vi "displayTest.vi"() -> ()   [LabVIEW 2010]
panel:
  in  "output cluster":T1
  out "display":T2={"电压/V"=[220.214842, 220.567942, 0.0], "测量变量显示"={"number: 0 to 1"=0.0, "number: 0 to 1"=0.0, "number: 0 to 1"=0.0}, "测量变量显示 2"={"number: 0 to 1"=0.0, "number: 0 to 1"=0.0, "number: 0 to 1"=0.0}}
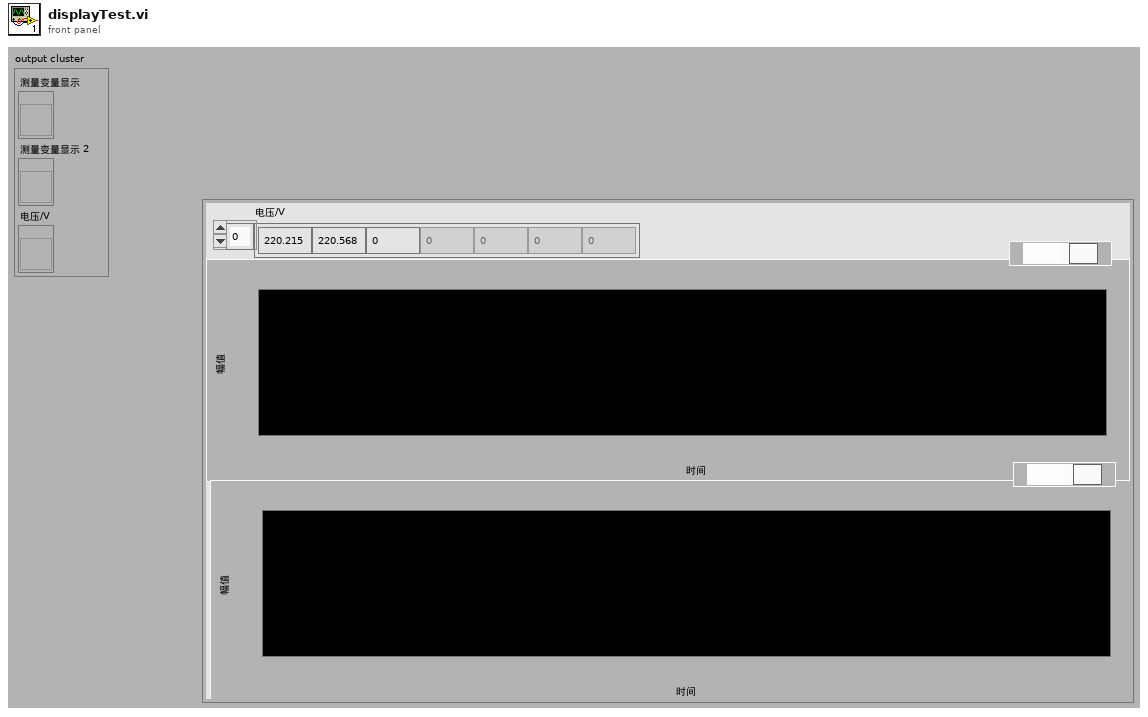
[diagram p1: front panel]
types:
  T1 = cluster{"测量变量显示":refnum<vi>, "测量变量显示 2":refnum<vi>, "电压/V":refnum<vi>}
  T2 = cluster{"电压/V":dbl[], "测量变量显示":cluster{"number: 0 to 1":dbl, "number: 0 to 1":dbl, "number: 0 to 1":dbl}, "测量变量显示 2":cluster{"number: 0 to 1":dbl, "number: 0 to 1":dbl, "number: 0 to 1":dbl}}
  T3 = cluster{"number: 0 to 1":dbl, "number: 0 to 1":dbl, "number: 0 to 1":dbl}[]
  T4 = typedef "OutputDataFormat.ctl" = cluster{"property":string, "dataIdentity":string, "value":string, "address":string, "timeStamp":string, "unit":string, "numID":i32, "VarableID":T5}
  T5 = typedef "VarableID.ctl" = enum16{"current", "power", "PF", "voltage"}
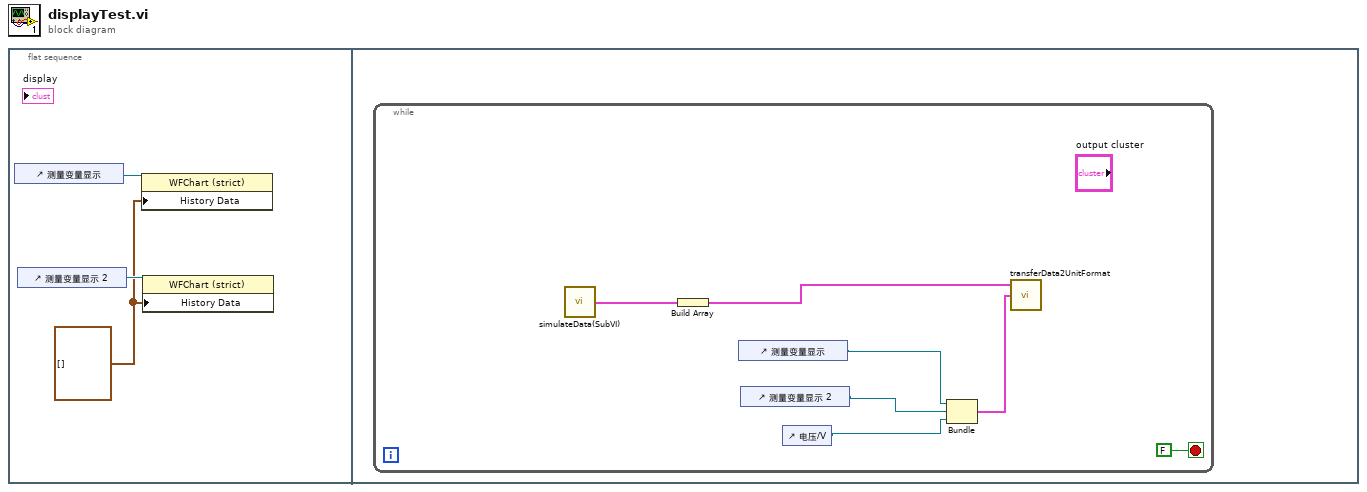
[diagram p0: block diagram]
diagram:
  n1 = flat-sequence {
    frame #0 {
      w1 = T3 [] ("History Data")
      n2 = control-ref of="测量变量显示"() -> (w3:refnum<vi>)
      n3 = control-ref of="测量变量显示 2"() -> (w2:refnum<vi>)
      n4 = property class="WFChart (strict)"(reference=w3, "History Data"=w1) -> ()  [unwired: 1 in, 2 out]
      n5 = property class="WFChart (strict)"(reference=w2, "History Data"=w1) -> ()  [unwired: 1 in, 2 out]
    }
    frame #1 {
      n6 = while {
        stop <- FALSE stop-if-true
        n7 = call "simulateData(SubVI).vi"() -> ("output cluster"=w5:T4)
        n8 = Build Array(w5) -> (w4:T4[])
        n9 = control-ref of="测量变量显示"() -> (w8:refnum<vi>)
        n10 = control-ref of="测量变量显示 2"() -> (w7:refnum<vi>)
        n11 = control-ref of="电压/V"() -> (w9:refnum<vi>)
        n12 = Bundle("测量变量显示"=w8, "测量变量显示 2"=w7, "电压/V"=w9) -> (w6:T1)  [unwired: 1 in]
        n13 = call "transferData2UnitFormat.vi"("displayRef"=w6, "Data"=w4) -> ()  [unwired: 3 in, 1 out]
      }
    }
  }
